vi "Read Msg Input.vi"(11 "Stopping Msg in":refnum<class "Stopping Msg.lvclass">) -> (2 "Msg Input":refnum<class "Msg Input.lvclass">)   [LabVIEW 2020, in "jettl.lvlib" / "Stopping jettl Msg.lvlib" / "Stopping Msg.lvlib" / "Stopping Msg.lvclass"]
doc: "jettl 6.12.1.94\nNathan Davis - Nathan Davis\nCopyright (c) 2026, Nathan Davis\nMIT"
uses:
  Stopping Msg.lvclass
  Msg Input/Msg Input.lvclass
  Stopping Msg.lvclass/Stopping Msg.ctl
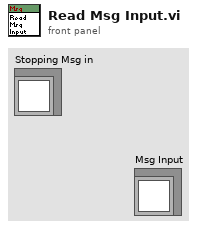
[diagram p1: front panel]
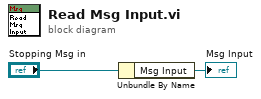
[diagram p0: block diagram]
diagram:
  n1 = Unbundle By Name("Stopping Msg in") -> ("Msg Input"=→"Msg Input":refnum<class "Msg Input.lvclass">)
